vi "PSTR-Process Frame.vi"(0 "Runtime in":T1 {"window" items=["None ", "Hanning", "Hamming", "Blackman-Harris", "Exact Blackman", "Blackman", "Flat Top", "4 Term B-Harris ", "7 Term B-Harris", "Low Sidelobe"]}, 5 "Override":bool, 7 "RejThr":dbl, 9 "data":dbl[](array[numeric]), 11 "error in (no error)":errorcluster) -> (4 "Runtime out":T1 {"window" items=["None ", "Hanning", "Hamming", "Blackman-Harris", "Exact Blackman", "Blackman", "Flat Top", "4 Term B-Harris ", "7 Term B-Harris", "Low Sidelobe"]}, 8 "reject":bool, 10 "done":bool, 13 "waveform":cluster{dbl, "dx":dbl, "Y":dbl[]}[](array[cluster]), 14 "status":string, 15 "error out":errorcluster)   [LabVIEW 2020]
uses:
  Typedefs/PSTR-Runtime Data.ctl
  epl-vi-lib/Signal Synthesis VIs/4th Generation/Classes/SignalManager/SignalManager.lvclass
  epl-vi-lib/Utility VIs/Conversion VIs/Create Waveform Cluster (1D).vi
  <vilib>/addons/Time Series Analysis/Correlation and Spectral Analysis.llb/TSA Welch (Array).vi
  <vilib>/addons/_Advanced Signal Processing/NI_AdvSigProcTSA.lvlib
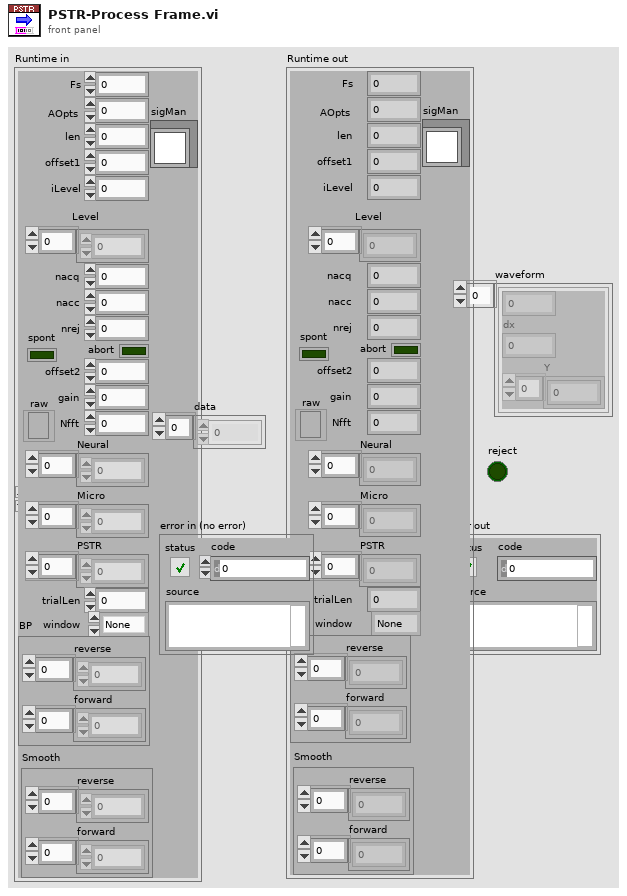
[diagram p1: front panel]
types:
  T1 = typedef "PSTR-Runtime Data.ctl" = cluster{"Fs":dbl, "AOpts":i32, "len":i32, "offset1":i32, "iLevel":i32, "Level":dbl[], "nacc":i32, "nrej":i32, "nacq":i32, "abort":bool, "offset2":i32, "gain":dbl, "Nfft":i32, "Neural":dbl[], "Micro":dbl[], "raw":refnum<file>, "spont":bool, "PSTR":dbl[], "trialLen":i32, "window":u16, "BP":cluster{"reverse":dbl[], "forward":dbl[]}, "Smooth":cluster{"reverse":dbl[], "forward":dbl[]}, "sigMan":refnum<class "SignalManager.lvclass">}
  T2 = cluster{"window":u16, "length":i32, "overlap (%)":dbl}
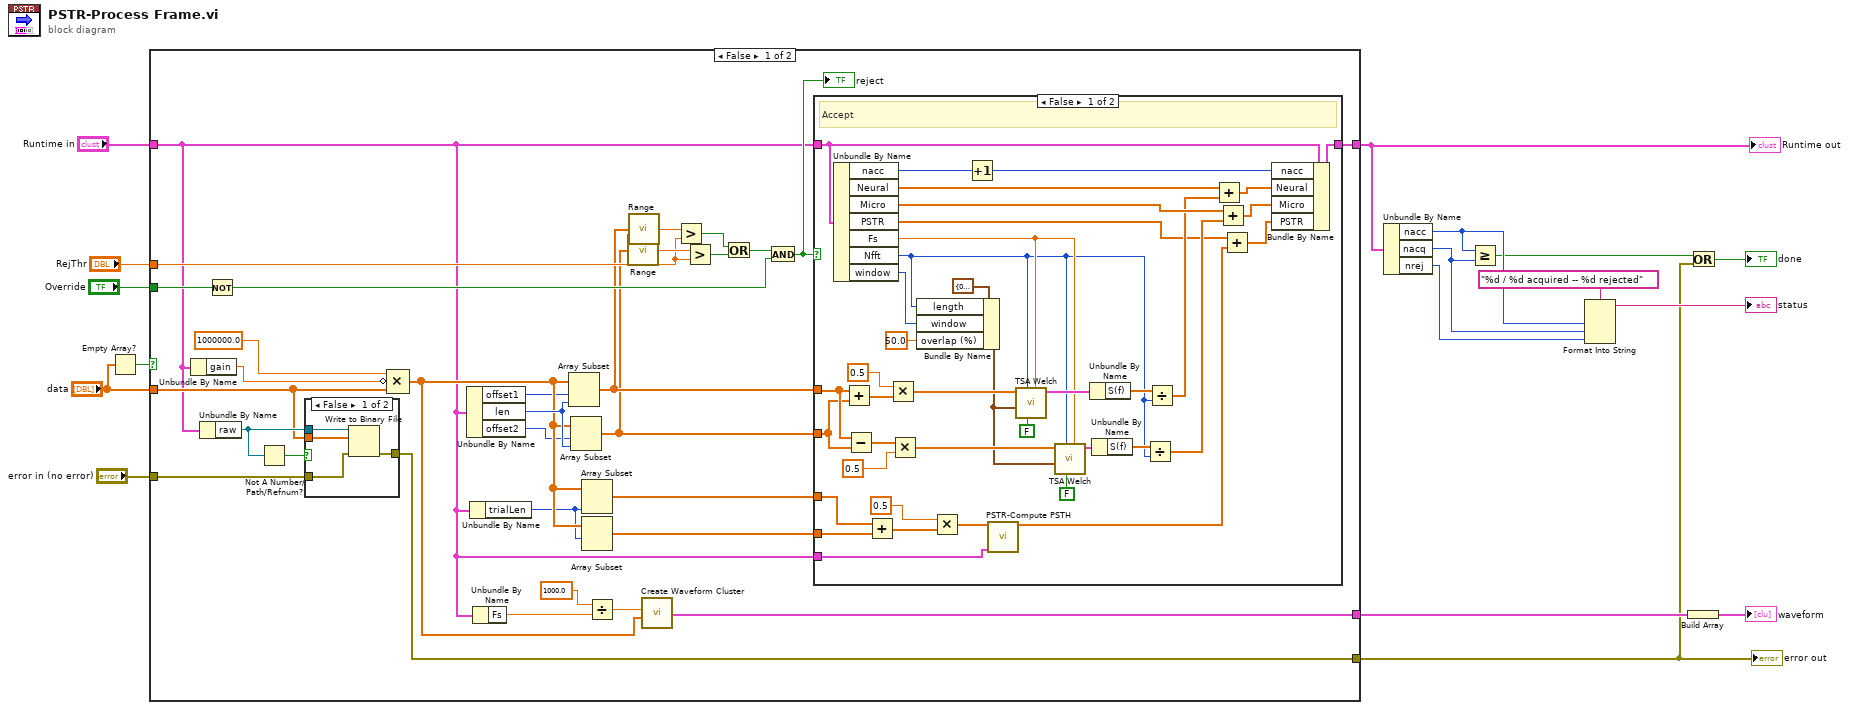
[diagram p0: block diagram]
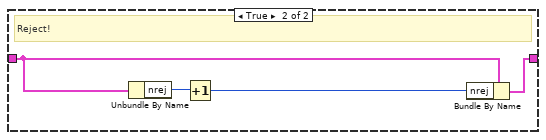
[diagram p3: hidden frame]
diagram:
  n1 = Empty Array?(array="data") -> (empty?=w4:bool)
  n2 = case shown="False" w4 {
    tunnel: [w46 _] -> w10
    tunnel: "data" -> [w30 _]
    tunnel: "RejThr" -> [w40 _]
    tunnel: "Override" -> [w36 _]
    tunnel: "Runtime in" -> [w18 w97]
    tunnel: [w33 w97] -> w5
    tunnel: [w28 w98] -> w2
    tunnel: "error in (no error)" -> [w29 w98]
    frame False {
      n3 = Unbundle By Name(w18) -> ("gain"=w44:dbl)
      n4 = Unbundle By Name(w18) -> ("raw"=w31:refnum<file>)
      n5 = Not(x=w36) -> (.not. x?=w35:bool)
      n6 = Not A Number/Path/Refnum?(number/path/refnum=w31) -> (NaN/Path/Refnum?=w32:bool)
      n7 = case shown="False" w32 {
        tunnel: w31 -> [w52 _]
        tunnel: w30 -> [w51 _]
        tunnel: w29 -> [w50 w53]
        tunnel: [w49 w53] -> w28
        frame False {
          n8 = Write to Binary File(file (use dialog)=w52, data=w51, error in=w50) -> (error out=w49:errorcluster)  [unwired: 3 in, 2 out]
        }
        frame True {
        }
      }
      n9 = Compound Arithmetic op=MULTIPLY(1000000.0, invert w44, w30) -> (w25:dbl[])
      n10 = Unbundle By Name(w18) -> ("offset1"=w24:i32, "len"=w45:i32, "offset2"=w23:i32)
      n11 = Unbundle By Name(w18) -> ("trialLen"=w19:i32)
      n12 = Unbundle By Name(w18) -> ("Fs"=w20:dbl)
      n13 = Array Subset(array=w25, index=w24, length=w45) -> (w27:dbl[])
      n14 = Array Subset(array=w25, index=w23, length=w45) -> (w26:dbl[])
      n15 = Array Subset(array=w25, length=w19) -> (w22:dbl[])  [unwired: 1 in]
      n16 = Array Subset(array=w25, index=w19) -> (w21:dbl[])  [unwired: 1 in]
      n17 = Divide(x=1000.0, y=w20) -> (x/y=w47:dbl)
      n18 = call "Range.vi"("Array"=w26) -> ("Range"=w41:dbl)
      n19 = call "Range.vi"("Array"=w27) -> ("Range"=w42:dbl)
      n20 = call-poly "Create Waveform Cluster.vi"("dx"=w47, "Y"=w25) -> ("waveform cluster"=w46:cluster{dbl, "dx":dbl, "Y":dbl[]})  [unwired: 3 in]
      n21 = Greater?(x=w42, y=w40) -> (0:w39:bool)
      n22 = Greater?(x=w41, y=w40) -> (0:w38:bool)
      n23 = Or(x=w39, y=w38) -> (x .or. y?=w37:bool)
      n24 = And(x=w37, y=w35) -> (x .and. y?=w34:bool)
      "reject" <- w34
      n25 = case shown="False" w34 {
        tunnel: w18 -> [w90 w95]
        tunnel: [w88 w93] -> w33
        tunnel: w27 -> [w84 _]
        tunnel: w26 -> [w83 _]
        tunnel: w22 -> [w62 _]
        tunnel: w21 -> [w61 _]
        tunnel: w18 -> [w54 _]
        frame False {
          # "Accept"
          n26 = Unbundle By Name(w90) -> ("nacc"=w89:i32, "Neural"=w74:dbl[], "Micro"=w71:dbl[], "PSTR"=w60:dbl[], "Fs"=w78:dbl, "Nfft"=w65:i32, "window"=w56:u16)
          n27 = Add(x=w84, y=w83) -> (x+y=w92:dbl[])
          n28 = Subtract(x=w84, y=w83) -> (x-y=w86:dbl[])
          n29 = Add(x=w62, y=w61) -> (x+y=w64:dbl[])
          n30 = Multiply(x=0.5, y=w92) -> (x*y=w81:dbl[])
          n31 = Multiply(x=w86, y=0.5) -> (x*y=w80:dbl[])
          n32 = Bundle By Name(cluster=T2 {"window"=0, "length"=2048, "overlap (%)"=50.0} ("window info"), "length"=w65, "window"=w56, "overlap (%)"=50.0) -> (w75:T2)
          n33 = Multiply(x=0.5, y=w64) -> (x*y=w58:dbl[])
          n34 = Increment(x=w89) -> (x+1=w87:i32)
          n35 = call "PSTR-Compute PSTH.vi"("Signal in"=w58, "Runtime"=w54) -> ("Signal out"=w57:dbl[])  [unwired: 13 in]
          n36 = call-poly <vilib>:"TSA Welch.vi"("sampling rate"=w78, "dB on? (T)"=FALSE, "frequency bins"=w65, "window info"=w75, "Xt"=w81) -> ("PSD"=w82:cluster{"f0":dbl, "df":dbl, "S(f)":dbl[]})  [unwired: 5 in, 1 out]
          n37 = call-poly <vilib>:"TSA Welch.vi"("sampling rate"=w78, "dB on? (T)"=FALSE, "frequency bins"=w65, "window info"=w75, "Xt"=w80) -> ("PSD"=w72:cluster{"f0":dbl, "df":dbl, "S(f)":dbl[]})  [unwired: 5 in, 1 out]
          n38 = Unbundle By Name(w82) -> ("S(f)"=w69:dbl[])
          n39 = Unbundle By Name(w72) -> ("S(f)"=w68:dbl[])
          n40 = Divide(x=w68, y=w65) -> (x/y=w66:dbl[])
          n41 = Divide(x=w69, y=w65) -> (x/y=w67:dbl[])
          n42 = Add(x=w74, y=w67) -> (x+y=w73:dbl[])
          n43 = Add(x=w71, y=w66) -> (x+y=w70:dbl[])
          n44 = Add(x=w60, y=w57) -> (x+y=w59:dbl[])
          n45 = Bundle By Name(cluster=w90, "nacc"=w87, "Neural"=w73, "Micro"=w70, "PSTR"=w59) -> (w88:T1)
        }
        frame True {
          # "Reject!"
          n46 = Unbundle By Name(w95) -> ("nrej"=w96:i32)
          n47 = Increment(x=w96) -> (x+1=w94:i32)
          n48 = Bundle By Name(cluster=w95, "nrej"=w94) -> (w93:T1)
        }
      }
    }
    frame True {
    }
  }
  "error out" <- w2
  "Runtime out" <- w5
  n49 = Unbundle By Name(w5) -> ("nacc"=w17:i32, "nacq"=w13:i32, "nrej"=w12:i32)
  n50 = Greater Or Equal?(x=w17, y=w13) -> (x >= y?=w16:bool)
  n51 = Format Into String(format string="%d / %d acquired -- %d rejected", w17, w13, w12) -> (resulting string=→"status":string)  [unwired: 2 in, 1 out]
  n52 = Build Array(w10) -> (→"waveform":cluster{dbl, "dx":dbl, "Y":dbl[]}[])
  n53 = Or(x=w16, y=w2) -> (x .or. y?=→"done":bool)
